vi "Get Request Type.vi"(8 "error in (no error)":errorcluster, 11 "SetPersistentData in":refnum<class "SetPersistentData.lvclass">) -> (0 "error out":errorcluster, 2 "Request Type":string, 3 "SetPersistentData out":refnum<class "SetPersistentData.lvclass">)   [LabVIEW 2022 SP3, in "obs-websocket-lv.lvlib" / "SetPersistentData.lvclass"]
uses:
  SetPersistentData.lvclass
  SetPersistentData.lvclass/SetPersistentData.ctl
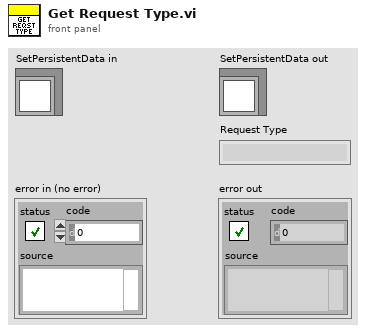
[diagram p1: front panel]
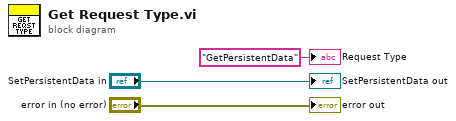
[diagram p0: block diagram]
diagram:
  "error out" <- "error in (no error)"
  "SetPersistentData out" <- "SetPersistentData in"
  "Request Type" <- "GetPersistentData" ("Request Type")
